vi "GetHumanInput.vi"(9 "Controller":dbl) -> (0 "Buttons":bool[](array[boolean]), 2 "POVs":i16[](array[numeric]), 3 "Axes":dbl[](array[numeric]))   [LabVIEW 2020]
uses:
  <vilib>/Rock Robotics/WPI/Utilities/WPI_GetSetVariantRefNum.vi
  <vilib>/Rock Robotics/Network Tables/NT Write Numeric Array.vi
  <vilib>/Rock Robotics/Network Tables/NT Write Boolean Array.vi
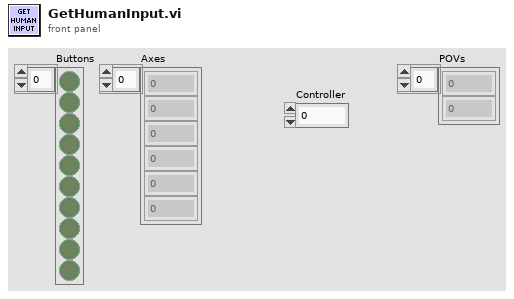
[diagram p1: front panel]
types:
  T1 = typedef "WPI_JoystickDevRef.ctl" = cluster{"Device":T2}
  T2 = typedef "WPI_JoystickDeviceEnum.ctl" = enum16{"USB 0", "USB 1", "USB 2", "USB 3", "USB 4", "USB 5"}
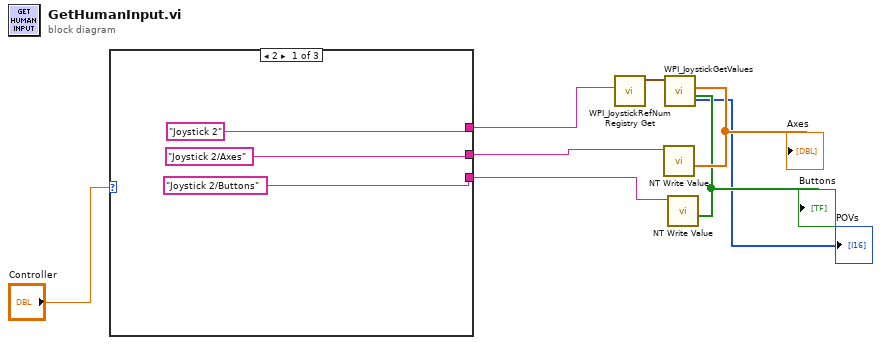
[diagram p0: block diagram]
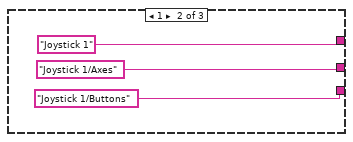
[diagram p2: hidden frame]
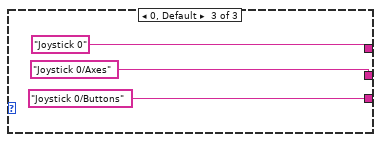
[diagram p3: hidden frame]
diagram:
  n1 = case shown="2" "Controller" {
    tunnel: ["Joystick 2/Buttons" ("Name") "Joystick 1/Buttons" ("Name") "Joystick 0/Buttons" ("Name")] -> w4
    tunnel: ["Joystick 2/Axes" ("Name") "Joystick 1/Axes" ("Name") "Joystick 0/Axes" ("Name")] -> w3
    tunnel: ["Joystick 2" ("refnum name") "Joystick 1" ("refnum name") "Joystick 0" ("refnum name")] -> w2
    frame 2 {
    }
    frame 1 {
    }
    frame 0, Default {
    }
  }
  n2 = call <vilib>:"WPI_JoystickRefNum Registry Get.vi"("refnum name"=w2) -> ("JoystickDevRef"=w8:T1)  [unwired: 1 in, 9 out]
  n3 = call <vilib>:"WPI_JoystickGetValues.vi"("JoystickDevRef"=w8) -> ("Buttons"=w6:bool[], "Axes"=w7:dbl[], "POVs"=→"POVs":i16[])  [unwired: 6 in, 2 out]
  "Buttons" <- w6
  "Axes" <- w7
  n4 = call-poly <vilib>:"NT Write Value.vi"("Numeric Array"=w7, "Name"=w3) -> ()  [unwired: 9 in, 1 out]
  n5 = call-poly <vilib>:"NT Write Value.vi"("Boolean Array"=w6, "Name"=w4) -> ()  [unwired: 9 in, 1 out]
